vi "LiCor_reader.vi"(8 "error in":errorcluster, 11 "VISA session in":refnum<visa-resource-name>="COM1") -> (0 "error out":errorcluster, 1 "read string":string, 2 "bytes read":u32, 3 "VISA session out":refnum<visa-resource-name>="COM1")   [LabVIEW 2010]
panel:
  # "LiCor Reader\n\nThis is a modular and small VI for reading data from the LiCor. It gets used in the LiCor_poller and LiCor_setting_manager VIs in order to retrieve data and clear buffers. For the most part, you should try to use those VIs."
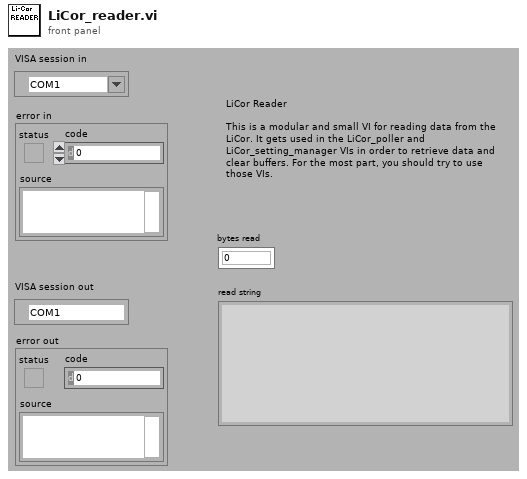
[diagram p1: front panel]
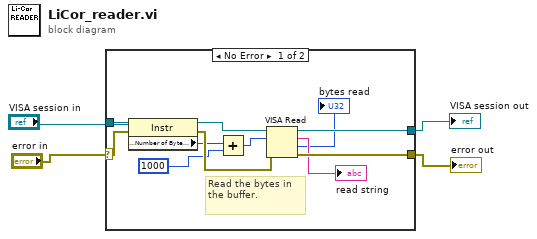
[diagram p0: block diagram]
diagram:
  n1 = case "Read bytes from port." shown="No Error" "error in" {
    selector: "error in" -> [w10 w17]
    tunnel: [w14 w17] -> w1
    tunnel: [w15 w16] -> w2
    tunnel: "VISA session in" -> [w11 w16]
    frame No Error {
      # "Read the bytes in the buffer."
      n2 = property class="Instr"(reference=w11, error in=w10) -> (reference out=w9:refnum<visa-resource-name>, error out=w8:errorcluster, "Serial Settings:Number of Bytes at Serial Port"=w7:u32)
      n3 = Add(x=w7, y=1000) -> (x+y=w6:u32)
      n4 = VISA Read(VISA resource name=w9, byte count=w6, error in (no error)=w8) -> (VISA resource name out=w15:refnum<visa-resource-name>, read buffer=→"read string":string, return count=→"bytes read":u32, error out=w14:errorcluster)
    }
    frame Error {
      # "Error occurred \nreading Bytes at \nSerial Port"
    }
  }
  "error out" <- w1
  "VISA session out" <- w2
